vi "Version.vi"() -> (1 "Version":string)   [LabVIEW 2023]
doc: "*-----------------------------------------------------\n* Author: SWatts\n*\n* VI Description: VI Constant that contains the version for this application, can be updated by Deploy if required\n* \n*\n* Error handling: All errors passed out\n*\n* Pre-condition: \n*\n* Post-condition: None\n*\n* Revision History:\n*\n* Rev Date Author Description \n* 01 30/04/2014 SWatts First issue\n*\n*-----------------------------------------------------"
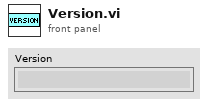
[diagram p1: front panel]
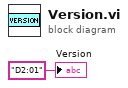
[diagram p0: block diagram]
diagram:
  "Version" <- "D2:01" ("Version")
